vi "Set PING))) Sensor.vi"(6 "PING))) sensor error (0)":i32, 8 "error in (no error)":errorcluster, 10 "PING)))":refnum<class "Parallax PING))).lvclass">, 11 "NI_Robotics_Starter Kit Host in":refnum<class "NI_Robotics_Starter Kit Host.lvclass">) -> (0 "error out":errorcluster, 3 "NI_Robotics_Starter Kit Host out":refnum<class "NI_Robotics_Starter Kit Host.lvclass">)   [LabVIEW 2017, in "NI_Robotics_Starter Kit Host.lvclass"]
uses:
  <vilib>/robotics/Starter Kit/Host Interface/NI_Robotics_Starter Kit Host.lvclass
  <instrlib>/Parallax PING)))/HAIOL/Parallax PING))).lvclass
  <vilib>/robotics/Starter Kit/Host Interface/NI_Robotics_Starter Kit Host.lvclass/NI_Robotics_Starter Kit Host.ctl
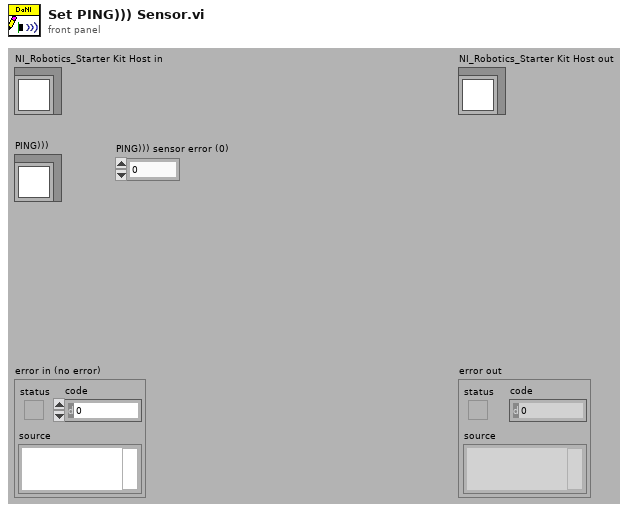
[diagram p1: front panel]
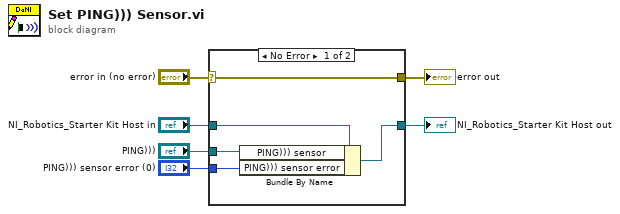
[diagram p0: block diagram]
diagram:
  n1 = case shown="No Error" "error in (no error)" {
    selector: "error in (no error)" -> [w11 w12]
    tunnel: [w11 w12] -> w5
    tunnel: [w9 w13] -> w3
    tunnel: "NI_Robotics_Starter Kit Host in" -> [w10 w13]
    tunnel: "PING)))" -> [w8 _]
    tunnel: "PING))) sensor error (0)" -> [w7 _]
    frame No Error {
      n2 = Bundle By Name(cluster=w10, "PING))) sensor"=w8, "PING))) sensor error"=w7) -> (w9:refnum<class "NI_Robotics_Starter Kit Host.lvclass">)
    }
    frame Error {
    }
  }
  "error out" <- w5
  "NI_Robotics_Starter Kit Host out" <- w3
